vi "hse-configuration_ReadStringKey.vi"(8 "error in (no error)":errorcluster, 9 "Key":string, 10 "Section":string, 11 "hse-config-ini in":refnum<class "hse-config-ini.lvclass">) -> (0 "error out":errorcluster, 2 "Value":string, 3 "hse-config-ini out":refnum<class "hse-config-ini.lvclass">)   [LabVIEW 2014, in "hse-config-ini.lvclass"]
doc: "Reads the string configuration value identified by <b>section</b> and <b>key</b> from the configuration object"
uses:
  hse-config-ini.lvclass
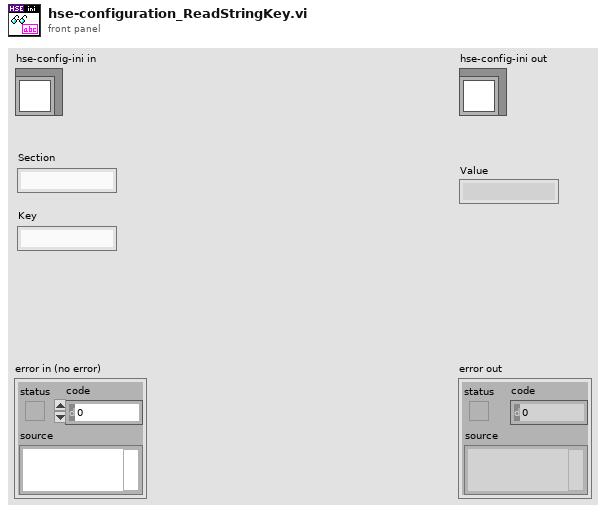
[diagram p1: front panel]
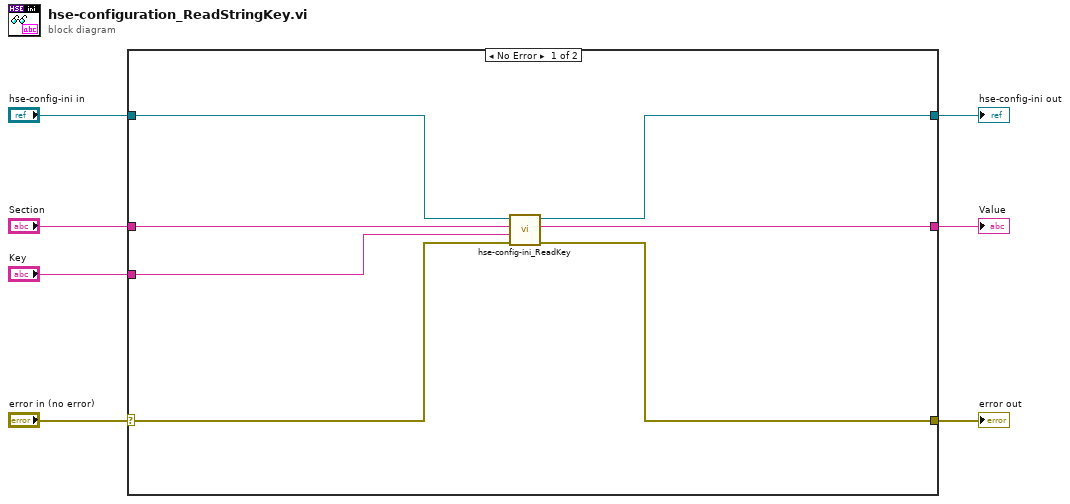
[diagram p0: block diagram]
diagram:
  n1 = case shown="No Error" "error in (no error)" {
    selector: "error in (no error)" -> [w10 w16]
    tunnel: [w8 w16] -> w6
    tunnel: "hse-config-ini in" -> [w14 w15]
    tunnel: [w13 w15] -> w4
    tunnel: "Section" -> [w12 _]
    tunnel: "Key" -> [w11 _]
    tunnel: [w9 _] -> w1
    frame No Error {
      n2 = call "hse-config-ini_ReadKey.vi"("error in (no error)"=w10, "Key"=w11, "Section"=w12, "hse-config-ini in"=w14) -> ("error out"=w8:errorcluster, "String"=w9:string, "hse-config-ini out"=w13:refnum<class "hse-config-ini.lvclass">)  [unwired: 5 in]
    }
    frame Error {
    }
  }
  "error out" <- w6
  "hse-config-ini out" <- w4
  "Value" <- w1
